vi "excel报表.vi"() -> ()   [LabVIEW 2014]
uses:
  <vilib>/addons/_office/_exclsub.llb/font.ctl
  <vilib>/Analysis/1siggen.llb/Ramp Pattern by Samples.vi
  <vilib>/Utility/NIReport.llb/NI_report.lvclass
  <vilib>/addons/_office/NI_ReportGenerationToolkit.lvlib
  <vilib>/Analysis/NI_AALBase.lvlib
panel:
  in  "report file path":path caption="报表文件路径"
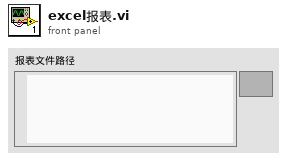
[diagram p1: front panel]
types:
  T1 = enum16{"maximized", "minimized", "normal", "no change"}
  T2 = typedef "NI_ReportGenerationToolkit.lvlib/font.ctl" = cluster{"font name":string, "font size":dbl, "bold":u16, "italic":u16, "underline":u16, "strike through":u16, "font color":u32}
  T3 = enum16{"Standard Report", "HTML", "Word", "Excel"}
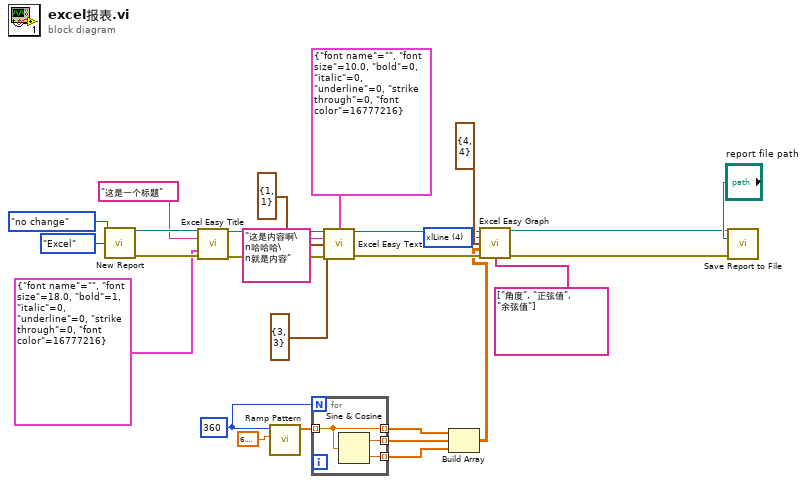
[diagram p0: block diagram]
diagram:
  w5 = 360 ("samples")
  w9 = 4 items=["xlColumnClustered"=51, "xlColumnStacked"=52, "xlColumnStacked100"=53, "xl3DColumnClustered"=54, "xl3DColumnStacked"=55, "xl3DColumnStacked100"=56, "xlBarClustered"=57, "xlBarStacked"=58, "xlBarStacked100"=59, "xl3DBarClustered"=60, "xl3DBarStacked"=61, "xl3DBarStacked100"=62, "xlLineStacked"=63, "xlLineStacked100"=64, "xlLineMarkers"=65, "xlLineMarkersStacked"=66, "xlLineMarkersStacked100"=67, "xlPieOfPie"=68, "xlPieExploded"=69, "xl3DPieExploded"=70, "xlBarOfPie"=71, "xlXYScatterSmooth"=72, "xlXYScatterSmoothNoMarkers"=73, "xlXYScatterLines"=74, "xlXYScatterLinesNoMarkers"=75, "xlAreaStacked"=76, "xlAreaStacked100"=77, "xl3DAreaStacked"=78, "xl3DAreaStacked100"=79, "xlDoughnutExploded"=80, "xlRadarMarkers"=81, "xlRadarFilled"=82, "xlSurface"=83, "xlSurfaceWireframe"=84, "xlSurfaceTopView"=85, "xlSurfaceTopViewWireframe"=86, "xlBubble"=15, "xlBubble3DEffect"=87, "xlStockHLC"=88, "xlStockOHLC"=89, "xlStockVHLC"=90, "xlStockVOHLC"=91, "xlCylinderColClustered"=92, "xlCylinderColStacked"=93, "xlCylinderColStacked100"=94, "xlCylinderBarClustered"=95, "xlCylinderBarStacked"=96, "xlCylinderBarStacked100"=97, "xlCylinderCol"=98, "xlConeColClustered"=99, "xlConeColStacked"=100, "xlConeColStacked100"=101, "xlConeBarClustered"=102, "xlConeBarStacked"=103, "xlConeBarStacked100"=104, "xlConeCol"=105, "xlPyramidColClustered"=106, "xlPyramidColStacked"=107, "xlPyramidColStacked100"=108, "xlPyramidBarClustered"=109, "xlPyramidBarStacked"=110, "xlPyramidBarStacked100"=111, "xlPyramidCol"=112, "xl3DColumn"=-4100, "xlLine"=4, "xl3DLine"=-4101, "xl3DPie"=-4102, "xlPie"=5, "xlXYScatter"=-4169, "xl3DArea"=-4098, "xlArea"=1, "xlDoughnut"=-4120, "xlRadar"=-4151] ("graph type (col clustered)")
  n1 = call <vilib>:"New Report.vi"("window state (normal)"=T1."no change", "report type"=T3."Excel") -> ("report out"=w25:refnum<class "NI_report.lvclass">, "error out"=w26:errorcluster)  [unwired: 12 in]
  n2 = call <vilib>:"Excel Easy Title.vi"("report in"=w25, "title"="这是一个标题", "font"=T2 {"font name"="", "font size"=18.0, "bold"=1, "italic"=0, "underline"=0, "strike through"=0, "font color"=16777216}, "error in (no error)"=w26) -> ("report out"=w22:refnum<class "NI_report.lvclass">, "error out"=w18:errorcluster)  [unwired: 9 in, 1 out]
  n3 = call-poly <vilib>:"Ramp Pattern.vi"("end"=6.283185307179586, "samples"=w5) -> ("Ramp Pattern"=w4:dbl[])  [unwired: 8 in, 1 out]
  n4 = for {
    N: w5 -> [_]
    tunnel: [w30] -> w8 mode=indexing
    tunnel: [w29] -> w7 mode=indexing
    tunnel: [w28] -> w3 mode=indexing
    tunnel: w4 -> [w28] mode=indexing
    n5 = Sine & Cosine(0:w28) -> (1:w30:dbl, 2:w29:dbl)
  }
  n6 = call <vilib>:"Excel Easy Text.vi"("report in"=w22, "font"=T2 {"font name"="", "font size"=10.0, "bold"=0, "italic"=0, "underline"=0, "strike through"=0, "font color"=16777216}, "text"="这是内容啊\n哈哈哈\n就是内容", "start (-1, -1)"=cluster{"row":i32, "column":i32} {"row"=1, "column"=1} ("start (0, 0)"), "end (-1, -1)"=cluster{"row":i32, "column":i32} {"row"=3, "column"=3}, "error in (no error)"=w18) -> ("report out"=w10:refnum<class "NI_report.lvclass">, "error out"=w14:errorcluster)  [unwired: 5 in, 3 out]
  n7 = Build Array(w3, w8, w7) -> (w2:dbl[][])
  n8 = call <vilib>:"Excel Easy Graph.vi"("report in"=w10, "graph type (col clustered)"=w9, "start (0, 0)"=cluster{"row":i32, "column":i32} {"row"=4, "column"=4}, "data"=w2, "error in (no error)"=w14, "row headers"=string[] ["角度", "正弦值", "余弦值"] ("column headers")) -> ("report out"=w11:refnum<class "NI_report.lvclass">, "error out"=w13:errorcluster)  [unwired: 8 in]
  n9 = call-dynamic "Save Report to File.vi"("report in"=w11, "report file path"="report file path", "error in (no error)"=w13) -> ()  [unwired: 11 in, 2 out]
